vi "temp.vi"() -> ()   [LabVIEW 2013]
panel:
  out "notification":variant
  out "Data":variant
  out "Command":string
  out "数值":i32
  in  "停止":bool
  in  "确定按钮":bool
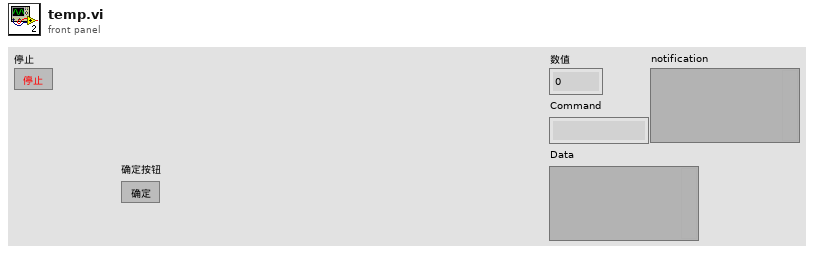
[diagram p1: front panel]
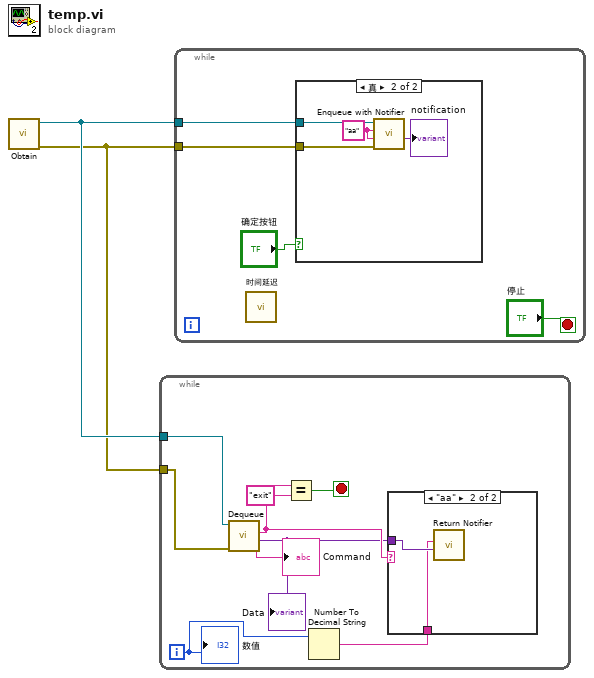
[diagram p0: block diagram]
diagram:
  n1 = call "Obtain.vi"() -> ("error out"=w1:errorcluster, "queue out"=w2:refnum<queue>)  [unwired: 9 in, 1 out]
  n2 = while {
    tunnel: w2 -> [w10]
    tunnel: w1 -> [w9]
    i -> [w4]
    stop <- w7 stop-if-true
    n3 = call "Dequeue.vi"("error in (no error)"=w9, "queue in"=w10) -> ("Data"=w5:variant, "Command"=w6:string)  [unwired: 5 in, 3 out]
    "Command" <- w6
    "Data" <- w5
    n4 = Equal?(x=w6, y="exit") -> (x = y?=w7:bool)
    n5 = Number To Decimal String(number=w4) -> (decimal integer string=w3:string)  [unwired: 1 in]
    n6 = case shown="\"aa\"" w6 {
      tunnel: w5 -> [_ w12]
      tunnel: w3 -> [_ w11]
      frame "假", Default {
      }
      frame "aa" {
        n7 = call "Return Notifier.vi"("Input Data"=w12, "Return Data"=w11) -> ()  [unwired: 8 in, 2 out]
      }
    }
    "数值" <- w4
  }
  n8 = while {
    tunnel: w2 -> [w15]
    tunnel: w1 -> [w14]
    stop <- "停止" stop-if-true
    n9 = call "时间延迟"() -> ()  [unwired: 11 in, 1 out]
    n10 = case shown="真" "确定按钮" {
      tunnel: w15 -> [_ w20]
      tunnel: w14 -> [_ w19]
      frame False {
      }
      frame True {
        w18 = "aa" ("Command")
        n11 = call "Enqueue with Notifier.vi"("error in"=w19, "Data"=w18, "Command"=w18, "command queue"=w20) -> ("notification"=→"notification":variant)  [unwired: 5 in, 2 out]
      }
    }
  }
